vi "Instr_SetPrivateData.vi"(8 "error in (no error)":errorcluster, 11 "KE236 in":refnum<class "KE236.lvclass">) -> (0 "error out":errorcluster, 3 "KE236 out":refnum<class "KE236.lvclass">)   [LabVIEW 2013, in "KE236.lvclass"]
uses:
  KE236.lvclass
  InstrumentSetup.vi
  KE236_CommandsGlobal.vi
  InstrControl.lvclass
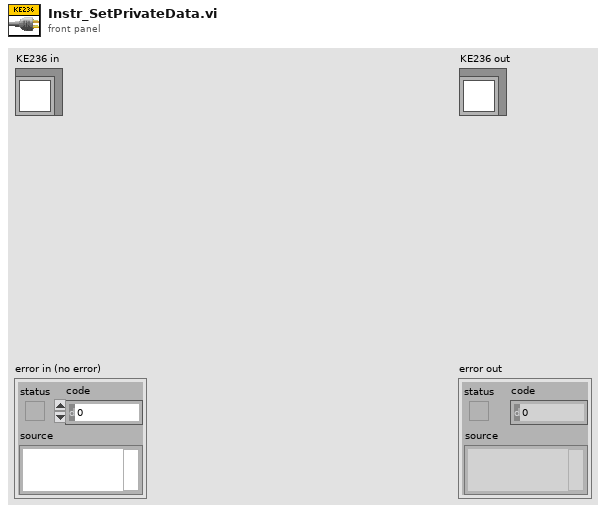
[diagram p1: front panel]
types:
  T1 = cluster{"current \ncompliance level":dbl, "compliance/\nmeasurement range (auto:0)":u16, "GPIB Address":string}
  T2 = cluster{"GPIB address":string, "Instrument name":string, "Instrument type":u16, "Command \"Reset\"":string, "Command \"Initialise\"":string, "Command \"Arm\"":string, "Command \"SetVolts\"":string, "Command \"Compliance?\"":string, "Command \"Standby\"":string, "Command \"Read Current\"":string}
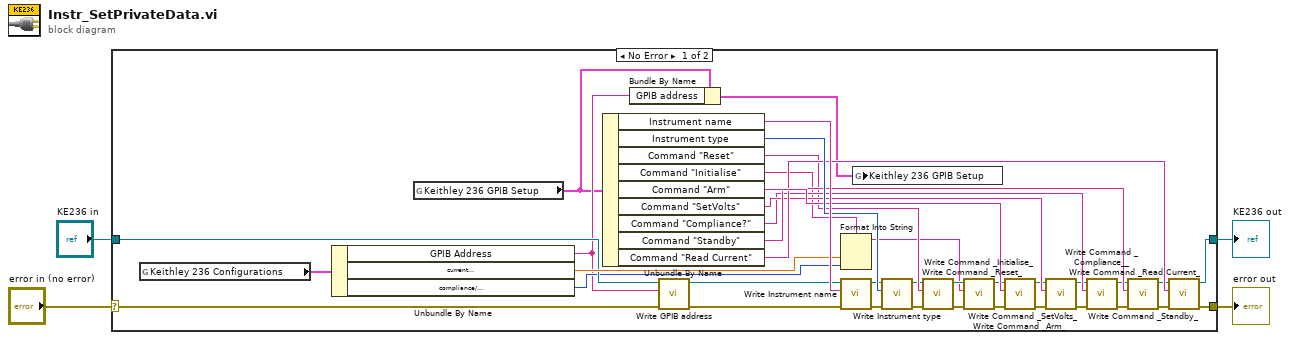
[diagram p0: block diagram]
diagram:
  n1 = case shown="No Error" "error in (no error)" {
    selector: "error in (no error)" -> [w25 w44]
    tunnel: [w9 w44] -> w1
    tunnel: "KE236 in" -> [w11 w43]
    tunnel: [w10 w43] -> w2
    frame No Error {
      n2 = global read "InstrumentSetup.vi" "Keithley 236 Configurations"() -> (w15:T1)
      n3 = Unbundle By Name(w15) -> ("GPIB Address"=w6:string, "current \ncompliance level"=w14:dbl, "compliance/\nmeasurement range (auto:0)"=w7:u16)
      n4 = global read "KE236_CommandsGlobal.vi" "Keithley 236 GPIB Setup"() -> (w5:T2)
      n5 = Unbundle By Name(w5) -> ("Instrument name"=w42:string, "Instrument type"=w41:u16, "Command \"Reset\""=w35:string, "Command \"Initialise\""=w13:string, "Command \"Arm\""=w40:string, "Command \"SetVolts\""=w37:string, "Command \"Compliance?\""=w36:string, "Command \"Standby\""=w38:string, "Command \"Read Current\""=w39:string)
      n6 = Bundle By Name(cluster=w5, "GPIB address"=w6) -> (w8:T2)
      n7 = call-dynamic "Write GPIB address.vi"("error in (no error)"=w25, "GPIB address"=w6, "InstControl in"=w11) -> ("error out"=w24:errorcluster, "InstControl out"=w34:refnum<class "KE236.lvclass">)  [unwired: 7 in]
      n8 = Format Into String(format string=w13, w14, w7) -> (resulting string=w12:string)  [unwired: 2 in, 1 out]
      n9 = call-dynamic "Write Instrument name.vi"("error in (no error)"=w24, "Instrument name"=w42, "InstControl in"=w34) -> ("error out"=w23:errorcluster, "InstControl out"=w33:refnum<class "KE236.lvclass">)  [unwired: 7 in]
      n10 = global write "KE236_CommandsGlobal.vi" "Keithley 236 GPIB Setup"(w8) -> ()
      n11 = call-dynamic "Write Instrument type.vi"("error in (no error)"=w23, "Instrument type"=w41, "InstControl in"=w33) -> ("error out"=w22:errorcluster, "InstControl out"=w32:refnum<class "KE236.lvclass">)  [unwired: 7 in]
      n12 = call-dynamic "Write Command _Reset_.vi"("error in (no error)"=w22, "Command \"Reset\""=w35, "SupplyControl in"=w32) -> ("error out"=w21:errorcluster, "SupplyControl out"=w31:refnum<class "KE236.lvclass">)  [unwired: 7 in]
      n13 = call-dynamic "Write Command _Initialise_.vi"("error in (no error)"=w21, "Command \"Initialise\""=w12, "SupplyControl in"=w31) -> ("error out"=w20:errorcluster, "SupplyControl out"=w30:refnum<class "KE236.lvclass">)  [unwired: 7 in]
      n14 = call-dynamic "Write Command _Arm_.vi"("error in (no error)"=w20, "Command \"Arm\""=w40, "SupplyControl in"=w30) -> ("error out"=w19:errorcluster, "SupplyControl out"=w29:refnum<class "KE236.lvclass">)  [unwired: 7 in]
      n15 = call-dynamic "Write Command _SetVolts_.vi"("error in (no error)"=w19, "Command \"SetVolts\""=w37, "SupplyControl in"=w29) -> ("error out"=w18:errorcluster, "SupplyControl out"=w28:refnum<class "KE236.lvclass">)  [unwired: 7 in]
      n16 = call-dynamic "Write Command _Compliance__.vi"("error in (no error)"=w18, "Command \"Compliance?\""=w36, "SupplyControl in"=w28) -> ("error out"=w17:errorcluster, "SupplyControl out"=w27:refnum<class "KE236.lvclass">)  [unwired: 7 in]
      n17 = call-dynamic "Write Command _Standby_.vi"("error in (no error)"=w17, "Command \"Standby\""=w38, "SupplyControl in"=w27) -> ("error out"=w16:errorcluster, "SupplyControl out"=w26:refnum<class "KE236.lvclass">)  [unwired: 7 in]
      n18 = call-dynamic "Write Command _Read Current_.vi"("error in (no error)"=w16, "Command \"Read Current\""=w39, "SupplyControl in"=w26) -> ("error out"=w9:errorcluster, "SupplyControl out"=w10:refnum<class "KE236.lvclass">)  [unwired: 7 in]
    }
    frame Error {
    }
  }
  "error out" <- w1
  "KE236 out" <- w2
